vi "funcaoAvaliacaoGoleiroBolaLongeArea.vi"(9 "balls":T1[](array[typedef]), 10 "Estado_Atual":T2(ring), 11 "IA State":T3={"our_robots"=[], "enemy_robots"=[], "balls"=[], "geometry"={"field_length"=0, "field_width"=0, "goal_width"=0, "goal_depth"=0, "center_circle_radius"=0, "defense_width"=0, "defense_depth"=0, "free_kick_from_defense_dist"=0, "penalty_spot_from_field_line_dist"=0, "penalty_line_from_spot_dist"=0, "half_moon_depth"=0, "half_moon_width"=0}, "IA Judge"={"stage"="", "command"="", "our_goalie_id"=0.0, "enemy_goalie_id"=0.0, "command enum"=enum."Halt", "Time"=enum."Azul"}, "Received Timestamp"=timestamp(0 s since 1904-01-01), "Events"={"Touch"=FALSE, "id touch"=0.0, "Ball out of \nVision"=FALSE, "Ball inside \nGoalie area"=FALSE, "Robot not responding"=FALSE, "Robots responding status"=[1.0, 1.0, 1.0, 1.0, 1.0, 1.0], "Enemy Ball \nPossession"=FALSE, "Id ini Possession"=0.0, "Ball Possesion"=FALSE, "Id Possesion"=0.0, "Ball at\nour goal side"=FALSE, "Ball at\ntouchline"=FALSE, "Ball at\nenemy goal side"=FALSE}}) -> (3 "Estado_Novo":T2(ring))   [LabVIEW 2018]
uses:
  Core/AI Input.ctl
  Core/AI Robot.ctl
  Intel/Functions Enum.ctl
  Intel/AttackerStates.ctl
  Path Planning/RRT/PathDests.ctl
  Path Planning/RRT/PathDest.ctl
  Core/AI Ball.ctl
  Core/Field Size.ctl
  Core/AI Judge.ctl
  Intel/Command Enum.ctl
  Util/Events/Events.ctl
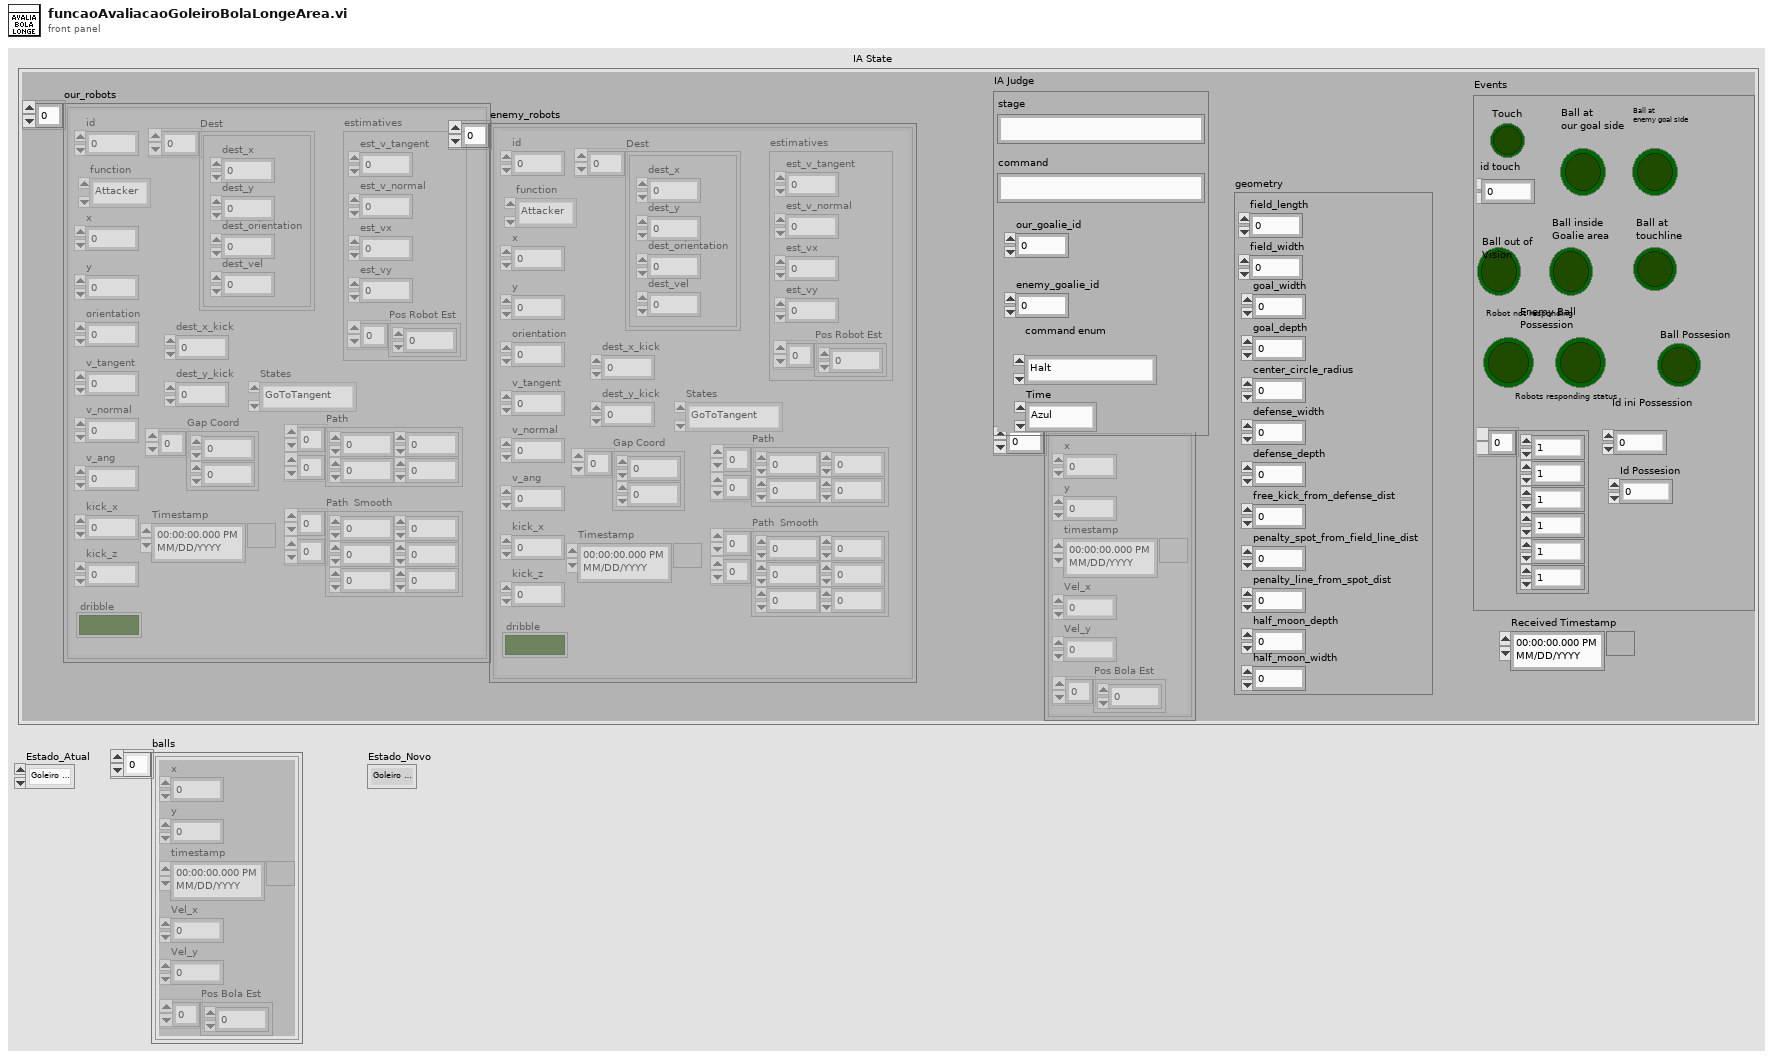
[diagram p1: front panel]
types:
  T1 = typedef "AI Ball.ctl" = cluster{"x":dbl, "y":dbl, "timestamp":timestamp, "Vel_x":dbl, "Vel_y":dbl, "Pos Bola Est":dbl[]}
  T2 = enum16{"Goleiro fora da área", "Alinhar com a bola", "Alinhar com a trave", "Rotacionar", "Aproximar-se da bola", "Posicionar-se na frente da bola"}
  T3 = typedef "AI Input.ctl" = cluster{"our_robots":T4[], "enemy_robots":T4[], "balls":T1[], "geometry":T9, "IA Judge":T10, "Received Timestamp":timestamp, "Events":T12}
  T4 = typedef "AI Robot.ctl" = cluster{"id":u32, "function":T5, "x":dbl, "y":dbl, "orientation":dbl, "v_tangent":dbl, "v_normal":dbl, "v_ang":dbl, "kick_x":dbl, "kick_z":dbl, "dribble":bool, "Timestamp":timestamp, "estimatives":cluster{"est_v_tangent":dbl, "est_v_normal":dbl, "est_vx":dbl, "est_vy":dbl, "Pos Robot Est":dbl[]}, "dest_x_kick":dbl, "dest_y_kick":dbl, "Gap Coord":dbl[], "States":T6, "Path ":dbl[][], "Path  Smooth":dbl[][], "Dest":T7}
  T5 = typedef "Functions Enum.ctl" = enum16{"Attacker", "Goalie", "Defender", "Striker", "Goto 0", "Dummy", "Kicker", "ZigZag"}
  T6 = typedef "AttackerStates.ctl" = enum16{"Pass", "GoToTangent", "BallGetting", "GoToKick", "Rotate anti-clockwise", "Rotate Clockwise", ""}
  T7 = typedef "PathDests.ctl" = T8[]
  T8 = typedef "PathDest.ctl" = cluster{"dest_x":dbl, "dest_y":dbl, "dest_orientation":dbl, "dest_vel":dbl}
  T9 = typedef "Field Size.ctl" = cluster{"field_length":u32, "field_width":u32, "goal_width":u32, "goal_depth":u32, "center_circle_radius":u32, "defense_width":u32, "defense_depth":u32, "free_kick_from_defense_dist":u32, "penalty_spot_from_field_line_dist":u32, "penalty_line_from_spot_dist":u32, "half_moon_depth":u32, "half_moon_width":u32}
  T10 = typedef "AI Judge.ctl" = cluster{"stage":string, "command":string, "our_goalie_id":dbl, "enemy_goalie_id":dbl, "command enum":T11, "Time":enum16{"Azul", "Amarelo"}}
  T11 = typedef "Command Enum.ctl" = enum16{"Halt", "Stop", "Force Start", "PKA Normal Start", "Prepare Kickoff Ally", "PKE Normal Start", "Prepare Kickoff Enemy", "Prepare Penalty Ally", "PPA Normal Start", "Prepare Penalty Enemy", "PPE Normal Start", "Ball Placement Enemy Up", "Ball Placement Enemy Down", "Ball Placement Ally Up", "Ball Placement Ally Mid", "Ball Placement Ally Down", "Indirect Free Enemy", "Indirect Free Ally", "Timeout Enemy", "Timeout Ally", "Goal Enemy", "Goal Ally", "Normal Half Time", "Extra Time Break", "Extra Half Time", "None", "Post Game"}
  T12 = typedef "Events.ctl" = cluster{"Touch":bool, "id touch":dbl, "Ball out of \nVision":bool, "Ball inside \nGoalie area":bool, "Robot not responding":bool, "Robots responding status":dbl[], "Enemy Ball \nPossession":bool, "Id ini Possession":dbl, "Ball Possesion":bool, "Id Possesion":dbl, "Ball at\nour goal side":bool, "Ball at\ntouchline":bool, "Ball at\nenemy goal side":bool}
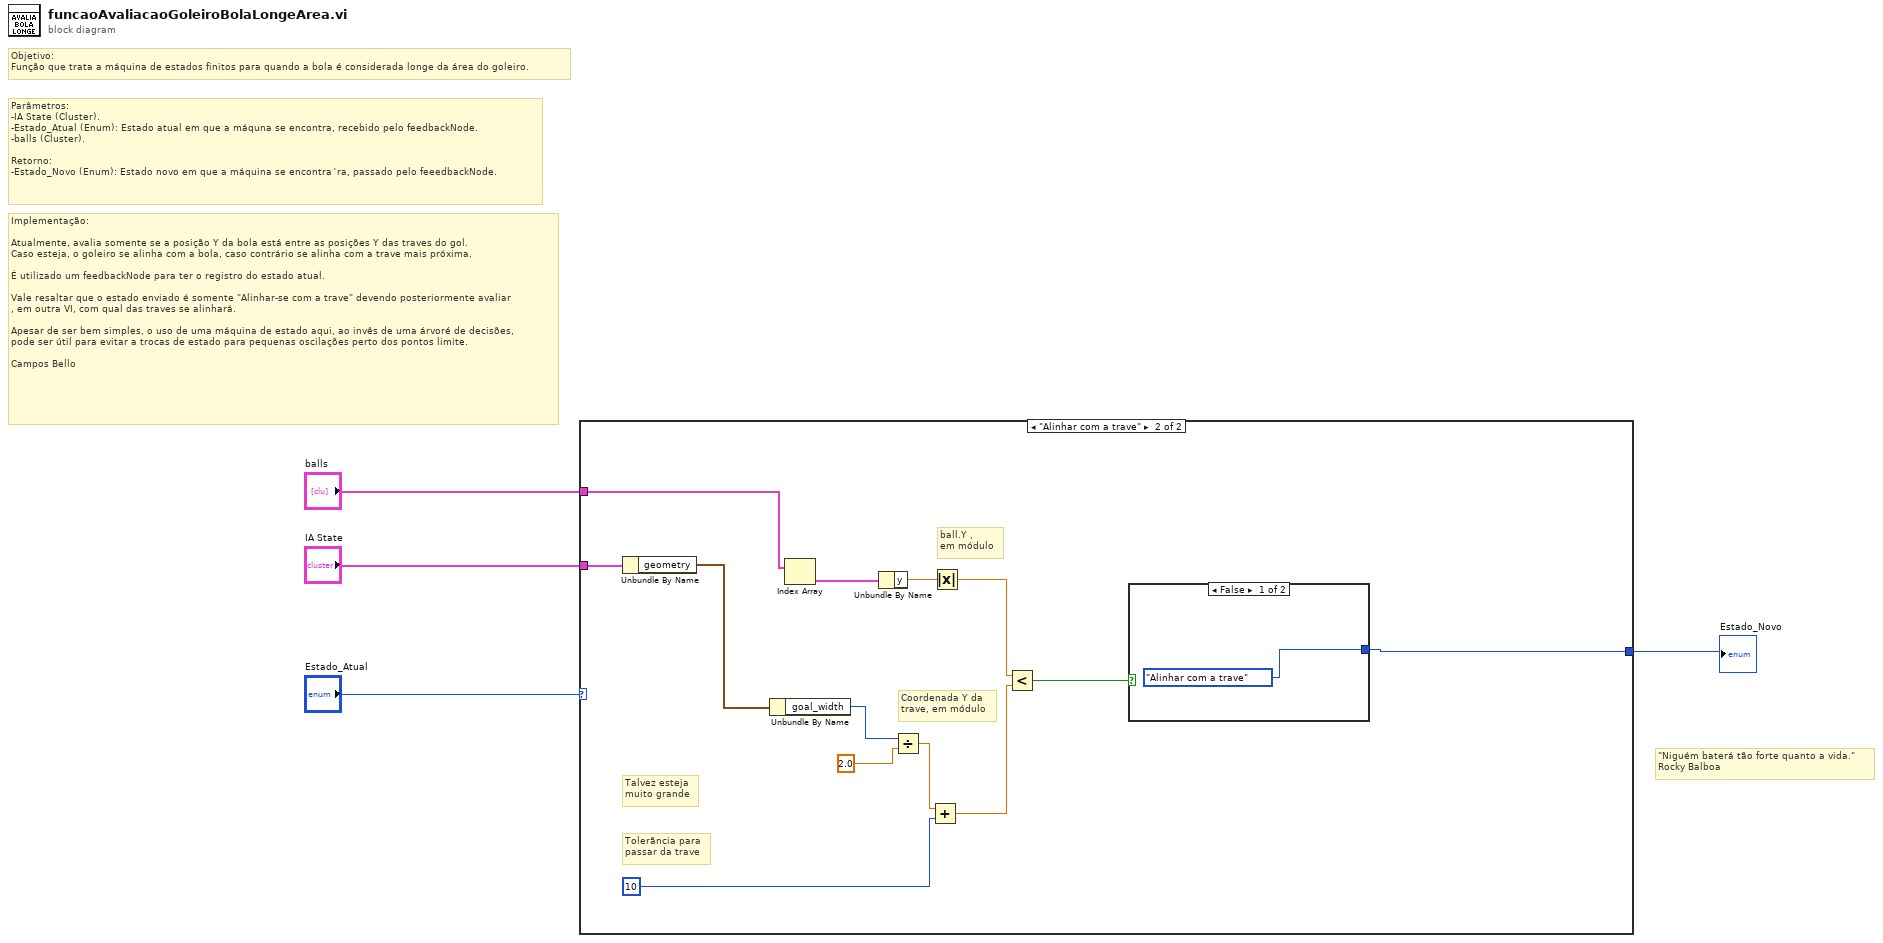
[diagram p0: block diagram]
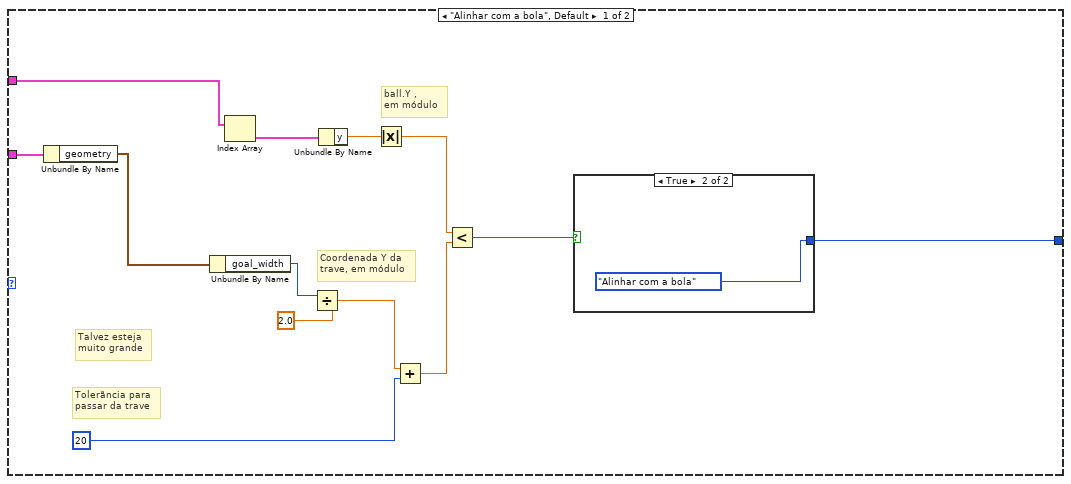
[diagram p2: hidden frame]
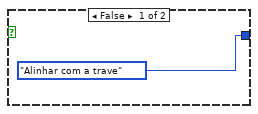
[diagram p3: hidden frame]
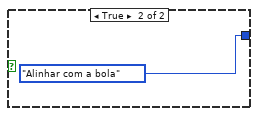
[diagram p4: hidden frame]
diagram:
  # "\"Niguém baterá tão forte quanto a vida.\"\nRocky Balboa"
  # "Parâmetros:\n-IA State (Cluster).\n-Estado_Atual (Enum): Estado atual em que a máquna se encontra, recebido pelo feedbackNode.\n-balls (Cluster).\n\nRetorno:\n-Estado_Novo (Enum): Estado novo em que a máquina se encontra´ra, passado pelo feeedbackNode."
  # "Implementação:\n\nAtualmente, avalia somente se a posição Y da bola está entre as posições Y das traves do gol.\nCaso esteja, o goleiro se alinha com a bola, caso contrário se alinha com a trave mais próxima.\n\nÉ utilizado um feedbackNode para ter o registro do estado atual.\n\nVale resaltar que o estado enviado é somente \"Alinhar-se com a trave\" devendo posteriormente avaliar\n, em outra VI, com qual das traves se alinhará.\n\nApesar de ser bem simples, o uso de uma máquina de estado aqui, ao invês de uma árvoré de decisões, \npode ser útil para evitar a trocas de estado para pequenas oscilações perto dos pontos limite.\n\nCampos Bello"
  # "Objetivo:\nFunção que trata a máquina de estados finitos para quando a bola é considerada longe da área do goleiro."
  n1 = case shown="\"Alinhar com a trave\"" "Estado_Atual" {
    tunnel: "IA State" -> [w17 w25]
    tunnel: [w9 w24] -> w2
    tunnel: "balls" -> [w5 w20]
    frame "Alinhar com a bola", Default {
      # "ball.Y ,\nem módulo"
      # "Coordenada Y da \ntrave, em módulo"
      # "Talvez esteja \nmuito grande"
      # "Tolerãncia para \npassar da trave"
      n2 = Unbundle By Name(w17) -> ("geometry"=w16:T9)
      n3 = Unbundle By Name(w16) -> ("goal_width"=w14:u32)
      n4 = Index Array(array=w5) -> (element=w13:T1)  [unwired: 1 in]
      n5 = Divide(x=w14, y=2.0) -> (x/y=w8:dbl)
      n6 = Unbundle By Name(w13) -> ("y"=w12:dbl)
      n7 = Absolute Value(x=w12) -> (abs(x)=w11:dbl)
      n8 = Add(x=w8, y=20) -> (x+y=w6:dbl)
      n9 = Less?(x=w11, y=w6) -> (x < y?=w10:bool)
      n10 = case shown="True" w10 {
        tunnel: [T2."Alinhar com a trave" ("Estado_Atual") T2."Alinhar com a bola" ("Estado_Atual")] -> w9
        frame False {
        }
        frame True {
        }
      }
    }
    frame "Alinhar com a trave" {
      # "Coordenada Y da \ntrave, em módulo"
      # "ball.Y ,\nem módulo"
      # "Talvez esteja \nmuito grande"
      # "Tolerãncia para \npassar da trave"
      n11 = Unbundle By Name(w25) -> ("geometry"=w32:T9)
      n12 = Unbundle By Name(w32) -> ("goal_width"=w30:u32)
      n13 = Index Array(array=w20) -> (element=w29:T1)  [unwired: 1 in]
      n14 = Unbundle By Name(w29) -> ("y"=w28:dbl)
      n15 = Divide(x=w30, y=2.0) -> (x/y=w22:dbl)
      n16 = Add(x=w22, y=10) -> (x+y=w21:dbl)
      n17 = Absolute Value(x=w28) -> (abs(x)=w27:dbl)
      n18 = Less?(x=w27, y=w21) -> (x < y?=w26:bool)
      n19 = case shown="False" w26 {
        tunnel: [T2."Alinhar com a trave" ("Estado_Atual") T2."Alinhar com a bola" ("Estado_Atual")] -> w24
        frame False {
        }
        frame True {
        }
      }
    }
  }
  "Estado_Novo" <- w2
